vi "Get as JSON string (pretty).vi"(8 "error in (no error)":errorcluster, 10 "Name Array":string[](array[string]), 11 "JSON Value in":refnum<class "JSON Value.lvclass">) -> (0 "error out":errorcluster, 2 "String":string)   [LabVIEW 2011, in "JSON Value.lvclass"]
uses:
  JSON Value.lvclass
panel:
  out "JSON Value out":refnum<class "JSON Value.lvclass">
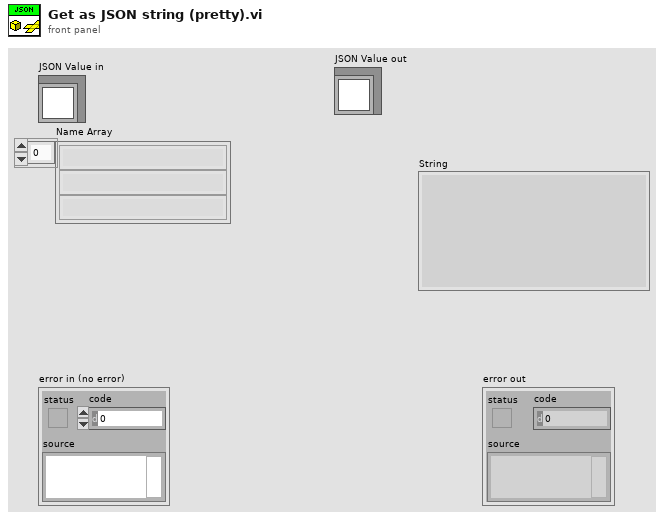
[diagram p1: front panel]
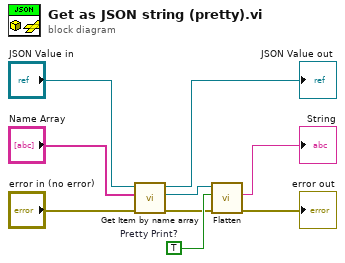
[diagram p0: block diagram]
diagram:
  w9 = TRUE  # Pretty Print?
  n1 = call "Get Item by name array.vi"("error in (no error)"="error in (no error)", "Name Array"="Name Array", "JSON Value In"="JSON Value in") -> ("error out"=w2:errorcluster, "Value"=w4:refnum<class "JSON Value.lvclass">, "JSON Value Out"=→"JSON Value out":refnum<class "JSON Value.lvclass">)  [unwired: 5 in, 1 out]
  n2 = call-dynamic "Flatten.vi"("error in (no error)"=w2, "Pretty Print?"=w9, "JSON Value in"=w4) -> ("error out"=→"error out":errorcluster, "String"=→"String":string)  [unwired: 7 in]
